vi "Scratchpad.vi"() -> ()   [LabVIEW 2020, in "FlexBlocks.lvlib"]
uses:
  FlexBlocks.lvlib
panel:
  out "error out":errorcluster
  out "Connection Path":path
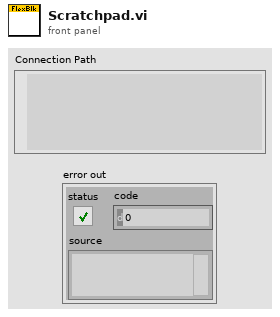
[diagram p1: front panel]
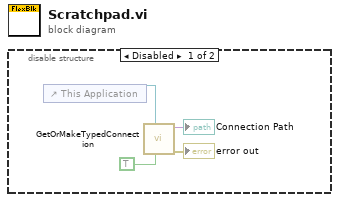
[diagram p0: block diagram]
diagram:
  n1 = disable-structure shown="Disabled" {
    frame Disabled {
      n2 = control-ref of="This Application"() -> (w4:refnum<vi>)
      n3 = call "GetOrMakeTypedConnection.vi"("Force Update? (F)"=TRUE, 7:w4) -> ("error out"=→"error out":errorcluster, "Connection"=→"Connection Path":variant)  [unwired: 7 in, 1 out]
    }
    frame Enabled {
    }
  }
